vi "Freq_block_Z.vi"(2 "w0":dbl=1.0 format="%#_13g", 3 "q_input":dbl[](array[numeric])=[915.3955183085, 84.33546198759, -358.8100229269, -15.56872770464, 872.6860692726]) -> (0 "al  fitness":dbl[](array[numeric]), 1 "q_output":dbl[](array[numeric]))   [LabVIEW 2015]
uses:
  <vilib>/Analysis/Matrix/Datatypes/RealMatrix.ctl
  <vilib>/Utility/file.llb/Read Delimited Spreadsheet (DBL).vi
  <vilib>/Analysis/Matrix/Numeric/Conversions/Array To Matrix - RA2.vi
  <vilib>/Analysis/Matrix/Numeric/Conversions/Matrix To Array - RM.vi
  <vilib>/Analysis/Matrix/Numeric/Conversions/Array To Matrix - RA.vi
  <vilib>/Analysis/baseanly.llb/Real Inverse Matrix.vi
  <vilib>/Analysis/Matrix/Numeric/Multiply/Multiply - RM,RM.vi
  <vilib>/Analysis/Matrix/NI_Matrix.lvlib
  <vilib>/Analysis/NI_AALBase.lvlib
panel:
  out "s? t:f":dbl[][](array[numeric])
  out "x+y":dbl[][](array[numeric])
  out "Array":bool[](array[boolean])
  out "weight":dbl
  out "Omega":dbl[][](array[numeric])
  out "gamma":dbl
  out "beta":dbl[](array[numeric])
  out "alpha":dbl
  out "q_bar":T1
  out "sumB":dbl[](array[numeric])
  out "finalB":dbl[](array[numeric])
  out "finalA":dbl[][](array[numeric])
  out "sumA":T1
  out "one constraint":dbl[](array[numeric])
  out "Nc":i32
  out "all constraints":dbl[][](array[numeric])
  out "size(s)":i32[](array[numeric])
  in  "Cnstraints path":path=path "D:/OneDrive/COURSES/LAB/2.LABVIEW_CODE/simulation/data/Freqconstraints.txt"
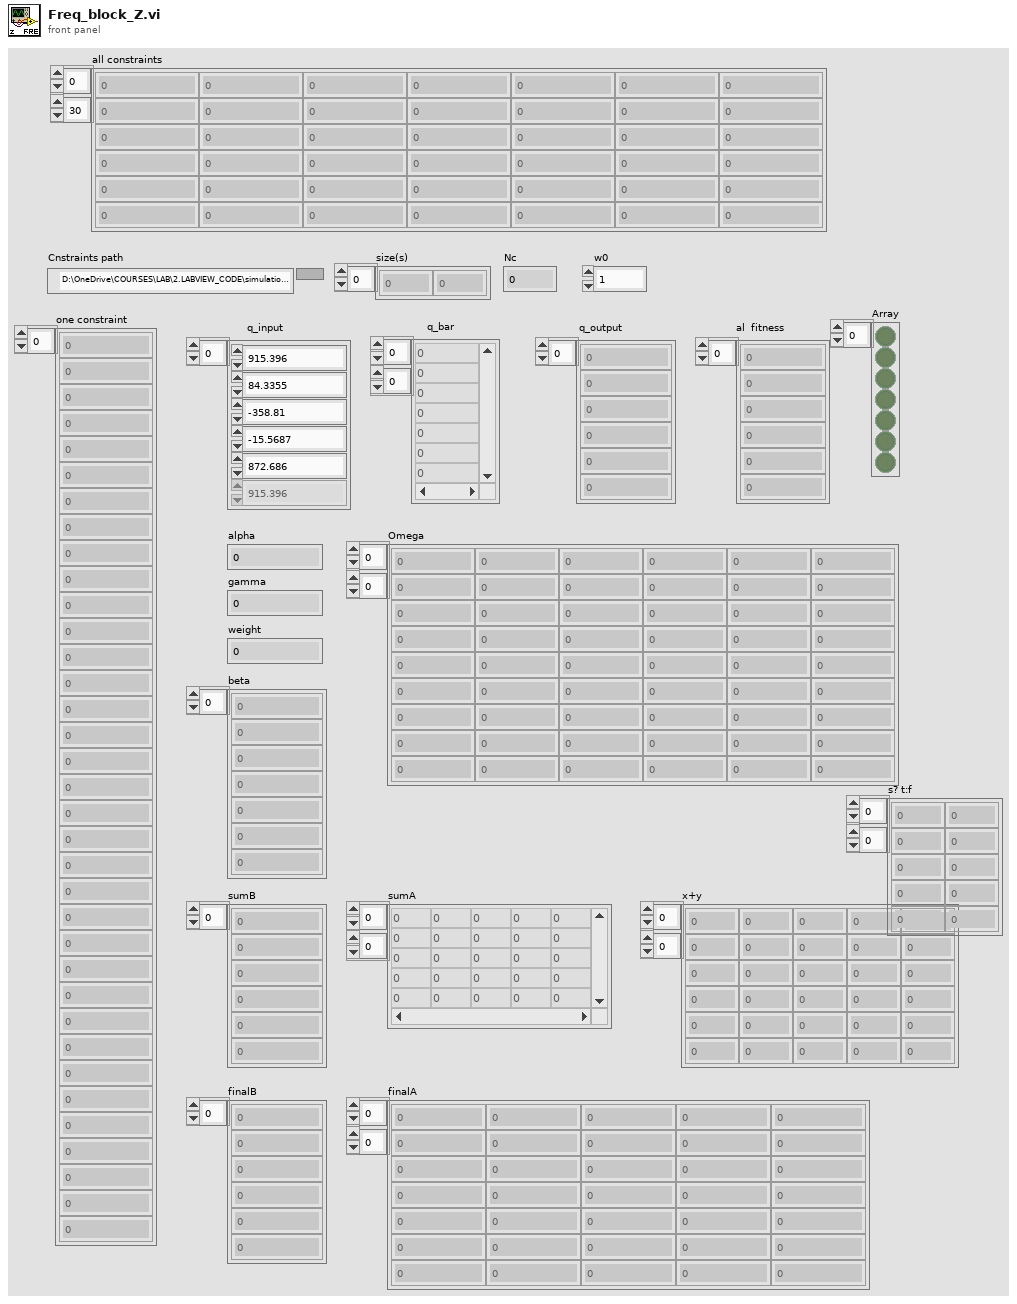
[diagram p1: front panel]
types:
  T1 = typedef "NI_Matrix.lvlib/RealMatrix.ctl" = dbl[][]
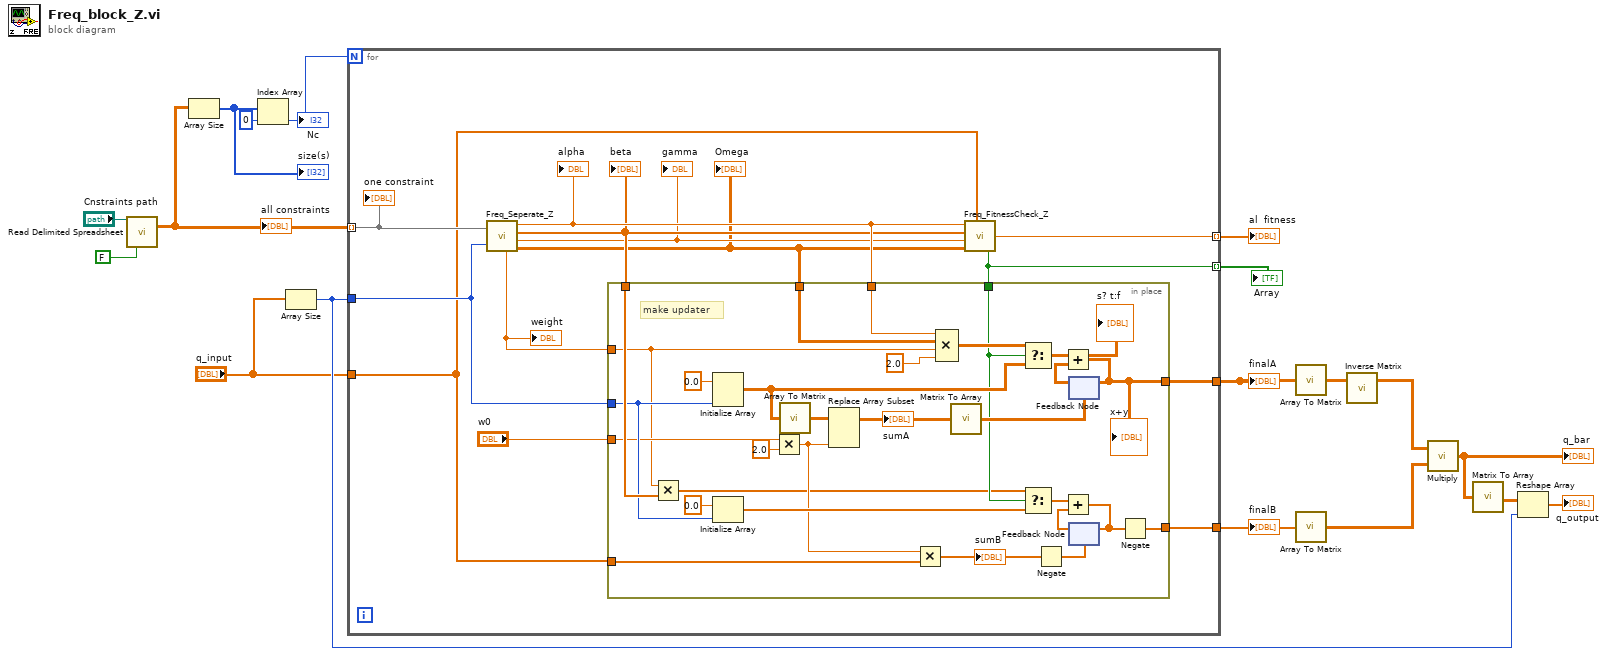
[diagram p0: block diagram]
diagram:
  n1 = call-poly <vilib>:"Read Delimited Spreadsheet.vi"("file path (dialog if empty)"="Cnstraints path", "transpose? (F)"=FALSE) -> ("all rows"=w14:dbl[][])  [unwired: 8 in, 5 out]
  "all constraints" <- w14
  n2 = Array Size(array=w14) -> (size(s)=w16:i32[])
  "size(s)" <- w16
  n3 = Index Array(array=w16, index=0) -> (element=w13:i32)
  "Nc" <- w13
  n4 = Array Size(array="q_input") -> (size(s)=w3:i32)
  n5 = for {
    N: w13 -> [_]
    tunnel: w14 -> [w26] mode=indexing
    tunnel: "q_input" -> [w20]
    tunnel: [w28] -> w12 mode=indexing
    tunnel: [w31] -> w11
    tunnel: [w30] -> w8
    tunnel: w3 -> [w27]
    tunnel: [w19] -> w1 mode=indexing
    n6 = call "Freq_Seperate_Z.vi"("constraint"=w26, "Length"=w27) -> ("weight"=w21:dbl, "alpha"=w25:dbl, "beta"=w24:dbl[], "gamma"=w23:dbl, "Omega"=w22:dbl[][])  [unwired: 1 in]
    "alpha" <- w25
    "beta" <- w24
    "gamma" <- w23
    "Omega" <- w22
    "weight" <- w21
    n7 = call "Freq_FitnessCheck_Z.vi"("alpha"=w25, "beta"=w24, "gamma"=w23, "Omega"=w22, "q_input"=w20) -> ("fitness"=w28:dbl, ">0"=w19:bool)  [unwired: 1 in]
    n8 = in-place {
      in-place-border: [w60] -> w31
      in-place-border: w22 -> [w55]
      in-place-border: w25 -> [w54]
      in-place-border: w24 -> [w49]
      in-place-border: [w36] -> w30
      in-place-border: w27 -> [w44]
      in-place-border: w19 -> [w43]
      in-place-border: "w0" -> [w41]
      in-place-border: w20 -> [w38]
      in-place-border: w21 -> [w33]
      # "make updater"
      n9 = Multiply(x=w33, y=w49) -> (x*y=w34:dbl[])
      n10 = Initialize Array(0.0 ("element"), w44, w44) -> (w52:dbl[][])
      n11 = Initialize Array(0.0 ("element"), w44) -> (w46:dbl[])
      n12 = Multiply(x=w41, y=2.0 ("new diagonal/fill element")) -> (x*y=w39:dbl)
      n13 = call-poly <vilib>:"Array To Matrix.vi"("Real 2D Array"=w52) -> ("Real Matrix"=w57:T1)
      n14 = Replace Array Subset(array=w57, new element=w39) -> (w32:T1)  [unwired: 2 in]
      "sumA" <- w32
      n15 = Multiply(x=w39, y=w38) -> (x*y=w40:dbl[])
      "sumB" <- w40
      n16 = Compound Arithmetic op=MULTIPLY(w54, w55, w33, 2.0 ("new diagonal/fill element")) -> (w53:dbl[][])
      n17 = call-poly <vilib>:"Matrix To Array.vi"("Real Matrix"=w32) -> ("Real 2D Array"=w56:dbl[][])
      n18 = Select(t=w53, s=w43, f=w52) -> (s? t:f=w51:dbl[][])
      "s? t:f" <- w51
      n19 = Select(t=w34, s=w43, f=w46) -> (s? t:f=w48:dbl[])
      n20 = Negate(x=w40) -> (-x=w37:dbl[])
      n21 = feedback #1(w56) -> (w59:dbl[][])
      n22 = Add(x=w51, y=w59) -> (x+y=w60:dbl[][])
      "x+y" <- w60
      n23 = feedback-in #1(w60) -> ()
      n24 = feedback #2(w37) -> (w47:dbl[])
      n25 = Add(x=w48, y=w47) -> (x+y=w45:dbl[])
      n26 = feedback-in #2(w45) -> ()
      n27 = Negate(x=w45) -> (-x=w36:dbl[])
    }
    "one constraint" <- w26
  }
  "al  fitness" <- w12
  "finalA" <- w11
  "finalB" <- w8
  "Array" <- w1
  n28 = call-poly <vilib>:"Array To Matrix.vi"("Real 2D Array"=w11) -> ("Real Matrix"=w10:T1)
  n29 = call-poly <vilib>:"Array To Matrix.vi"("Real 1D Array"=w8) -> ("Real Matrix (Column Vector)"=w7:T1)
  n30 = call-poly <vilib>:"Inverse Matrix.vi"("Input Matrix"=w10) -> ("Inverse Matrix"=w9:T1)  [unwired: 1 in, 1 out]
  n31 = call-poly <vilib>:"Multiply.vi"("Real Matrix B"=w7, "Real Matrix A"=w9) -> ("A * B"=w6:T1)
  "q_bar" <- w6
  n32 = call-poly <vilib>:"Matrix To Array.vi"("Real Matrix"=w6) -> ("Real 2D Array"=w5:dbl[][])
  n33 = Reshape Array(w5, w3) -> (→"q_output":dbl[])
